vi "在线发送.vi"(6 "标志位":string, 7 "VISA资源名称":refnum<visa-resource-name>, 8 "错误输入（无错误）":errorcluster, 9 "结果":bool, 10 "中心点Y值":ext, 11 "中心点X值":ext) -> (0 "错误输出":errorcluster, 2 "完整帧":string, 3 "返回码":string)   [LabVIEW 2012]
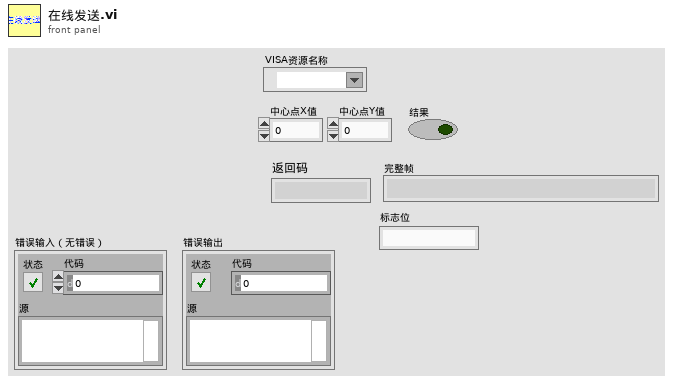
[diagram p1: front panel]
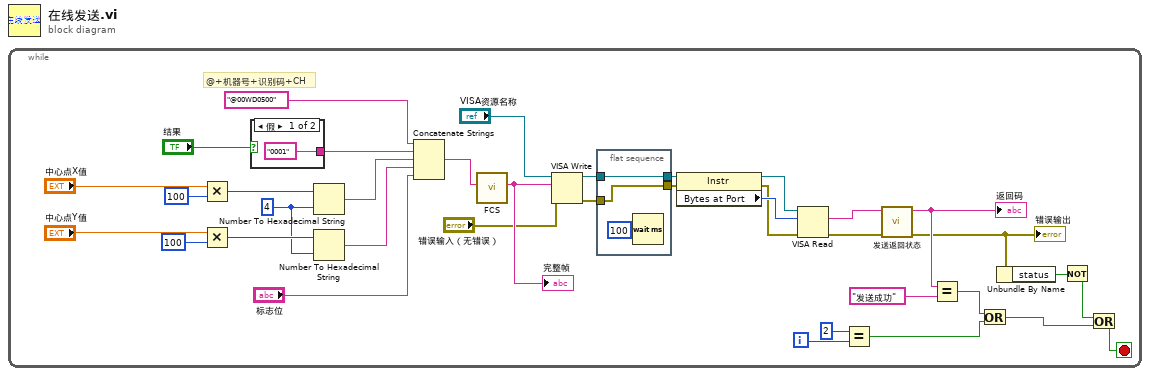
[diagram p0: block diagram]
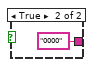
[diagram p2: hidden frame]
diagram:
  n1 = while {
    i -> [w12]
    stop <- w4 stop-if-true
    w20 = i16 4 ("宽度(-)")
    # "@+机器号+识别码+CH"
    n2 = Multiply ("乘")(x="中心点X值", y=100) -> (x*y=w22:i32)
    n3 = Multiply ("乘")(x="中心点Y值", y=100) -> (x*y=w21:i32)
    n4 = case shown="假" "结果" {
      tunnel: ["0001" ("发送命令") "0000" ("发送命令")] -> w17
      frame False {
      }
      frame True {
      }
    }
    n5 = Number To Hexadecimal String(1:w20, 2:w22) -> (0:w16:string)
    n6 = Number To Hexadecimal String(1:w20, 2:w21) -> (0:w15:string)
    n7 = Concatenate Strings("@00WD0500" ("发送命令"), w17, w16, w15, "标志位") -> (w14:string)
    n8 = call "FCS.vi"("发送命令"=w14) -> ("完整帧"=w35:string)  [unwired: 10 in]
    "完整帧" <- w35
    n9 = VISA Write(VISA resource name="VISA资源名称", write buffer=w35, error in (no error)="错误输入（无错误）") -> (VISA resource name out=w34:refnum<visa-resource-name>, error out=w32:errorcluster)  [unwired: 1 out]
    n10 = flat-sequence {
      tunnel: w34 -> [w42]
      tunnel: [w42] -> w33
      tunnel: w32 -> [w41]
      tunnel: [w41] -> w31
      frame #0 {
        n11 = Wait (ms)(milliseconds to wait=100) -> ()  [unwired: 1 out]
      }
    }
    n12 = property class="Instr"(reference=w33, error in=w31) -> (reference out=w37:refnum<visa-resource-name>, error out=w30:errorcluster, "Bytes at Port"=w36:u32)
    n13 = VISA Read(VISA resource name=w37, byte count=w36, error in (no error)=w30) -> (read buffer=w28:string, error out=w29:errorcluster)  [unwired: 2 out]
    n14 = Equal?(x=2, y=w12) -> (x = y?=w10:bool)
    n15 = call "发送返回状态.vi"("错误输入"=w29, "字符串"=w28) -> ("错误输出"=w6:errorcluster, "返回"=w9:string)  [unwired: 8 in]
    "返回码" <- w9
    "错误输出" <- w6
    n16 = Equal?(x=w9, y="发送成功") -> (x = y?=w7:bool)
    n17 = Or(x=w7, y=w10) -> (x .or. y?=w2:bool)
    n18 = Unbundle By Name(w6) -> ("status"=w5:bool)
    n19 = Not(x=w5) -> (.not. x?=w3:bool)
    n20 = Or(x=w3, y=w2) -> (x .or. y?=w4:bool)
  }
